vi "Close.vi"(8 "error in (no error)":errorcluster, 11 "Base Hardware in":refnum<class "Base Hardware.lvclass">) -> (0 "error out":errorcluster, 3 "Base Hardware out":refnum<class "Base Hardware.lvclass">)   [LabVIEW 2023, in "Abstract Hardware.lvlib" / "Base Hardware.lvclass"]
uses:
  Base Hardware.lvclass
  Base Hardware.lvclass/Base Hardware.ctl
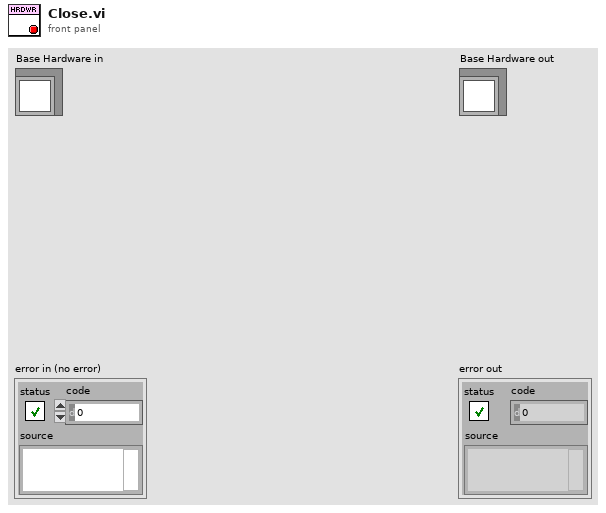
[diagram p1: front panel]
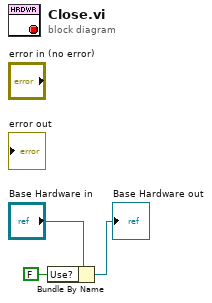
[diagram p0: block diagram]
diagram:
  n1 = Bundle By Name(cluster="Base Hardware in", "Use?"=FALSE) -> (→"Base Hardware out":refnum<class "Base Hardware.lvclass">)
